vi "New Bump Align Traj.vi"() -> ()   [LabVIEW 2025]
uses:
  Framework/Robot Global Data.vi
  <vilib>/Analysis/NI_AALPro.lvlib
  <vilib>/Rock Robotics/WPI/DriverStation/WPI_DriverStationAllianceInfo.ctl
  <vilib>/Analysis/coordinate.llb/2D Cartesian Coordinate Rotation (Scalar).vi
  bordeaux/Bordeaux/Types/Limits.ctl
  swerve-template/Type Definitions/Data/Robot Velocities.ctl
panel:
  out "th":dbl
  in  "Auto Data In":T2
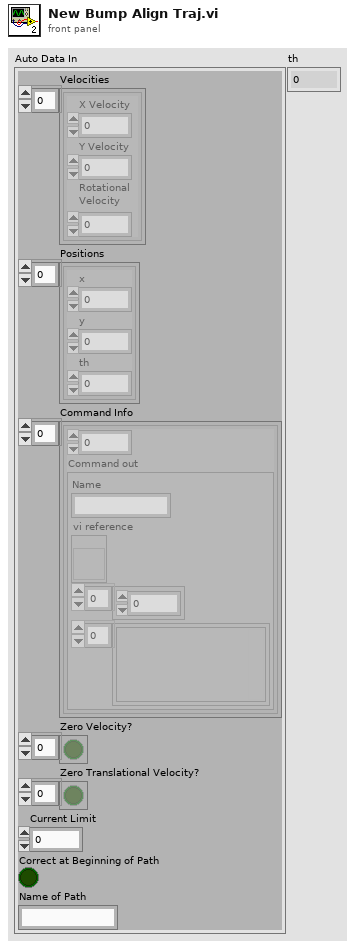
[diagram p1: front panel]
types:
  T1 = typedef "Robot Velocities.ctl" = cluster{"X Velocity":dbl, "Y Velocity":dbl, "Rotational \nVelocity":dbl}
  T2 = cluster{"Velocities":T1[], "Positions":cluster{"x":dbl, "y":dbl, "th":dbl}[], "Command Info":cluster{dbl, "Command out":cluster{"Name":string, "vi reference":refnum<vi>, i32[], variant[]}}[], "Zero Velocity?":bool[], "Zero Translational Velocity?":bool[], "Current Limit":dbl, "Correct at Beginning of Path":bool, "Name of Path":string}
  T3 = typedef "Limits.ctl" = cluster{"Velocity (fps)":dbl, "Accel (fps^2)":dbl, "Jerk (fps^3)":dbl, "StoopidFast (fps)":dbl}
  T4 = typedef "WPI_DriverStationAllianceInfo.ctl" = enum16{"Red", "Blue", "Invalid"}
  T5 = typedef "Segment Type.ctl" = enum16{"Accel Straight", "Const Straight", "Blend", "Circle", "Bezier"}
  T6 = cluster{"Segment Name":string, "Type":T5, "Traj Pos Points":cluster{"x":dbl, "y":dbl, "th":dbl}[], "Traj Vel Points":cluster{"V":dbl, "Omega":dbl, "V vector":cluster{"y":dbl, "x":dbl}}[], "Accel Index":i32, "Decel Index":i32}[]
  T7 = cluster{"Segment Name":string, "Type":T5, "Traj Pos Points":cluster{"x":dbl, "y":dbl, "th":dbl}[], "Traj Vel Points":cluster{"V":dbl, "Omega":dbl, "V vector":cluster{"y":dbl, "x":dbl}}[], "Accel Index":i32, "Decel Index":i32}
  T8 = cluster{"V":dbl, "Omega":dbl, "V vector":cluster{"y":dbl, "x":dbl}}[]
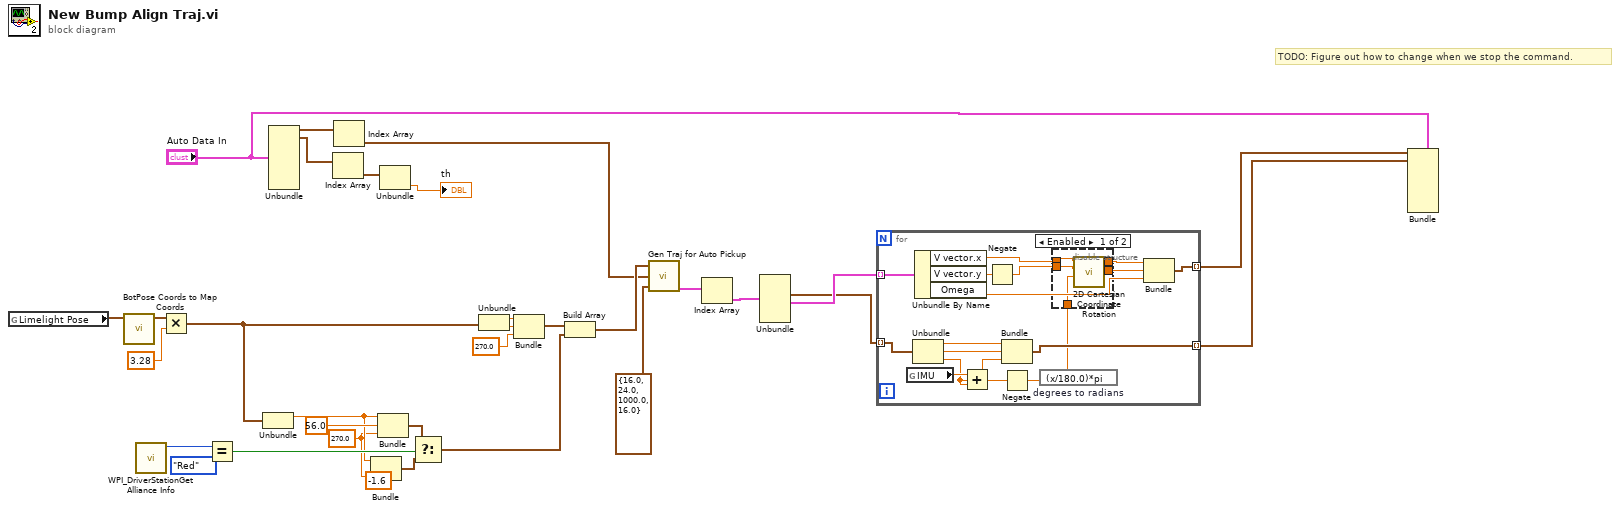
[diagram p0: block diagram]
diagram:
  w15 = 270.0
  # "TODO: Figure out how to change when we stop the command."
  n1 = global read "Robot Global Data.vi" "Limelight Pose"() -> (w28:cluster{"X":dbl, "Y":dbl})
  n2 = call "BotPose Coords to Map Coords.vi"("Point In"=w28) -> ("Point Out"=w27:cluster{dbl, dbl})  [unwired: 10 in]
  n3 = call <vilib>:"WPI_DriverStationGet Alliance Info.vi"() -> ("Alliance"=w22:T4)  [unwired: 6 in, 5 out]
  n4 = Multiply(x=w27, y=3.28) -> (x*y=w20:cluster{dbl, dbl})
  n5 = Equal?(x=w22, y=WPI_DriverStationAllianceInfo."Red") -> (x = y?=w18:bool)
  n6 = Unbundle(w20) -> (w16:dbl)  [unwired: 1 out]
  n7 = Unbundle("Auto Data In") -> ("Velocities"=w9:T1[], "Positions"=w3:cluster{"x":dbl, "y":dbl, "th":dbl}[])  [unwired: 6 out]
  n8 = Index Array(array=w3) -> (element=w2:cluster{"x":dbl, "y":dbl, "th":dbl})  [unwired: 1 in]
  n9 = Index Array(array=w9) -> (element=w8:T1)  [unwired: 1 in]
  n10 = Bundle(w16, -1.6, w15) -> (w13:cluster{dbl, dbl, dbl})  [unwired: 1 in]
  n11 = Bundle(w16, 56.0, w15) -> (w12:cluster{dbl, dbl, dbl})  [unwired: 1 in]
  n12 = Unbundle(w2) -> ("th"=→"th":dbl)  [unwired: 2 out]
  n13 = Select(t=w12, s=w18, f=w13) -> (s? t:f=w11:cluster{dbl, dbl, dbl})
  n14 = Unbundle(w20) -> (w25:dbl, w24:dbl)
  n15 = Bundle(w25, w24, 270.0) -> (w19:cluster{dbl, dbl, dbl})  [unwired: 1 in]
  n16 = Build Array(w19, w11) -> (w10:cluster{dbl, dbl, dbl}[])
  n17 = call "Gen Traj for Auto Pickup.vi"("Path Positions"=w10, "Robot Velocities"=w8, "Limits"=T3 {"Velocity (fps)"=16.0, "Accel (fps^2)"=24.0, "Jerk (fps^3)"=1000.0, "StoopidFast (fps)"=16.0}) -> ("Trajectory Data Out"=w32:T6)  [unwired: 1 in, 2 out]
  n18 = Index Array(array=w32) -> (element=w31:T7)  [unwired: 1 in]
  n19 = Unbundle(w31) -> ("Traj Pos Points"=w29:cluster{"x":dbl, "y":dbl, "th":dbl}[], "Traj Vel Points"=w30:T8)  [unwired: 4 out]
  n20 = for {
    tunnel: w30 -> [w49] mode=indexing
    tunnel: w29 -> [w46] mode=indexing
    tunnel: [w45] -> w5 mode=indexing
    tunnel: [w39] -> w6 mode=indexing
    n21 = global read "Robot Global Data.vi" "IMU"() -> (w44:dbl)
    n22 = Unbundle(w46) -> ("x"=w47:dbl, "y"=w48:dbl, "th"=w36:dbl)
    n23 = Unbundle By Name(w49) -> ("V vector.x"=w34:dbl, "V vector.y"=w43:dbl, "Omega"=w40:dbl)
    n24 = Add(x=w44, y=w36) -> (x+y=w37:dbl)
    n25 = Negate(x=w43) -> (-x=w42:dbl)
    n26 = Bundle("x"=w47, "y"=w48, w37) -> (w45:cluster{"x":dbl, "y":dbl, dbl})  [unwired: 1 in]
    n27 = Negate(x=w36) -> (-x=w38:dbl)
    n28 = expression code="(x/180.0)*pi" "degrees to radians"(w38) -> (w35:dbl)
    n29 = disable-structure shown="Enabled" {
      disable-tunnel: w34 -> [w54 w56]
      disable-tunnel: w42 -> [w53 w55]
      disable-tunnel: [w52 w56] -> w33
      disable-tunnel: [w51 w55] -> w41
      disable-tunnel: w35 -> [w50 _]
      frame Enabled {
        n30 = call-poly <vilib>:"2D Cartesian Coordinate Rotation.vi"("theta"=w50, "y"=w53, "x"=w54) -> ("y out"=w51:dbl, "x out"=w52:dbl)  [unwired: 6 in, 1 out]
      }
      frame Disabled {
      }
    }
    n31 = Bundle("x out"=w33, "y out"=w41, "Omega"=w40) -> (w39:cluster{"x out":dbl, "y out":dbl, "Omega":dbl})  [unwired: 1 in]
  }
  n32 = Bundle(cluster="Auto Data In", "Velocities"=w6, "Positions"=w5) -> ()  [unwired: 6 in, 1 out]
